vi "count rate.vi"() -> (2 "output waveform":waveform(i32), 3 "Counts per second":i32[](array[numeric])=[0, 39, 50, 53, 43, 50, 43, 47, 49, 37, 40, 55, 56, 54, 41, 52, 42, 50, 55, 55, 45, 36, 58, 52, 48, 47, 54, 50, 64, 44, 52, 51, 34, 52, 46, 42, 50, 45, 40, 42, 45, 40, 42, 59, 53, 48, 43, 37, 28, 32, 29, 31, 30, 44, 40, 33, 48, 33, 36, 38, 41, 31, 35, 37, 38, 40, 40, 22, 25, 37, 35, 33, 39, 39, 33, 33, 30, 28, 35, 32, 21, 45, 30, 25, 33, 21, 30, 28, 34, 17, 24, 19, 24, 27, 32, 30, 18, 28, 28, 22, 18, 23, 28, 33, 21, 18, 24, 20, 30, 26, 27, 17, 19, 22, 18, 21, 16, 20, 20, 19, 18, 22, 22, 22, 22, 22, 25, 24, 16, 20, 12, 21, 17, 24, 14, 24, 11, 13, 19, 21, 18, 13, 11, 13, 10, 15, 12, 12, 18, 12, 18, 18, 14, 11, 17, 16, 10, 11, 22, 18, 17, 10, 10, 10, 14, 17, 11, 8, 11, 13, 7, 10, 14, 13, 16, 13, 8, 9, 11, 10, 10, 4, 10, 10, 8, 13, 10, 9, 16, 13, 11, 10, 4, 7, 7, 8, 7, 6, 7, 10, 8, 9, 12, 13, 7, 11, 11, 0, 11, 9, 7, 6, 11, 10, 1, 11, 5, 4, 10, 9, 8, 5, 6, 11, 9, 8, 3, 10, 6, 7, 8, 7, 5, 7, 6, 8, 9, 9, 8, 9, 8, 6, 6, 10, 7, 4, 7, 8, 2, 9, 9, 10, 8, 7, 9, 3, 4, 7, 4, 5, 8, 4, 6, 6, 9, 3, 8, 8, 7, 5, 10, 4, 7, 2, 9, 9, 6, 3, 3, 4, 4, 2, 5, 3, 2, 4, 8, 8, 3, 5, 1, 6, 3, 1, 4, 5, 6, 7, 2, 5, 3, 3])   [LabVIEW 2014]
uses:
  <vilib>/Platform/TimedLoop/XDataNode/timing_clust.ctl
  <vilib>/Platform/TimedLoop/XDataNode/nitl_modes.ctl
  <vilib>/Platform/TimedLoop/XDataNode/wakeup.ctl
  <vilib>/Waveform/WDTFileIO.llb/ Write Waveform to File.vi
  <vilib>/Utility/file.llb/Write To Spreadsheet File (I64).vi
  <vilib>/platform/TimedLoop/XDataNode/XDataNode.xnode
  <vilib>/Platform/TimedLoop/XDataNode/XDNodeRunTimeDep.lvlib
panel:
  out "Waveform Graph":waveform(i32)(graph)
  in  "Period (ms)":i64=1000
  in  "Total time (sec)":i32=300
  out "counts per second":dbl(knob)=3.0 scale=0.0..100.0
  # "Demo count rate VI for Physics 434"
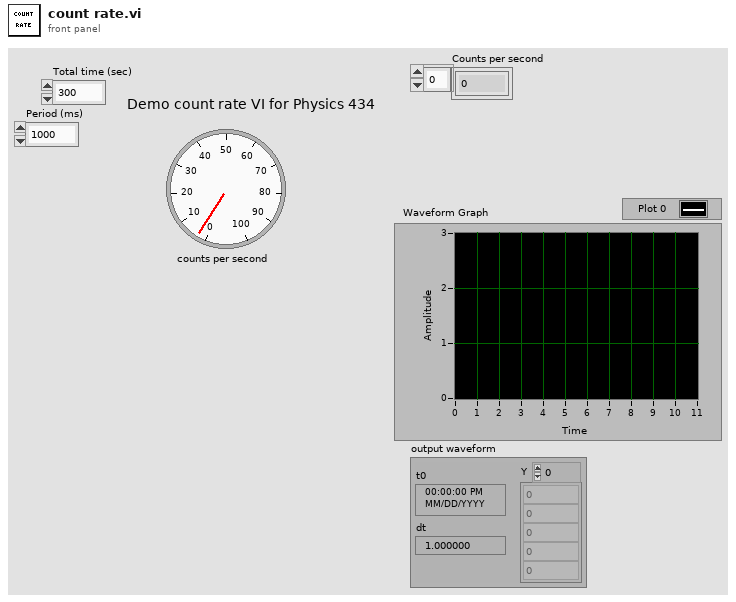
[diagram p1: front panel]
types:
  T1 = typedef "XDNodeRunTimeDep.lvlib/timing_clust.ctl" = cluster{"Expected End [f-1]":u64, "Actual End [f-1]":u64, "Finished Late? [f-1]":bool, "Expected End [i-1]":u64, "Actual End [i-1]":u64, "Finished Late? [i-1]":bool, "Expected Start [i]":u64, "Actual Start [i]":u64, "Expected Start [f]":u64, "Actual Start [f]":u64, "Source Name":string, "Structure Name":string, "Period":i64, "Deadline":i64, "Offset":i64, "Start":i64, "Priority":i32, "Timeout":i32, "Mode":T2, "Wakeup Reason":T3, "Error":errorcluster, "Source Type":string, "Secondary Source Type":string, "Global End Time":u64, "Global Start Time":u64, "Frame Duration":u64, "Iteration Duration":u64, "Assigned CPU":i32, "I/O Scan Engine Mode":u32}
  T2 = typedef "XDNodeRunTimeDep.lvlib/nitl_modes.ctl" = enum32{"No Change", "Process missed periods, maintain original phase", "Discard missed periods, maintain original phase", "Process missed periods, ignore original phase", "Discard missed periods, ignore original phase"}
  T3 = typedef "XDNodeRunTimeDep.lvlib/wakeup.ctl" = enum32{"Normal", "Aborted", "Asynchronous wakeup", "Timing source error", "Timed loop error", "Timeout"}
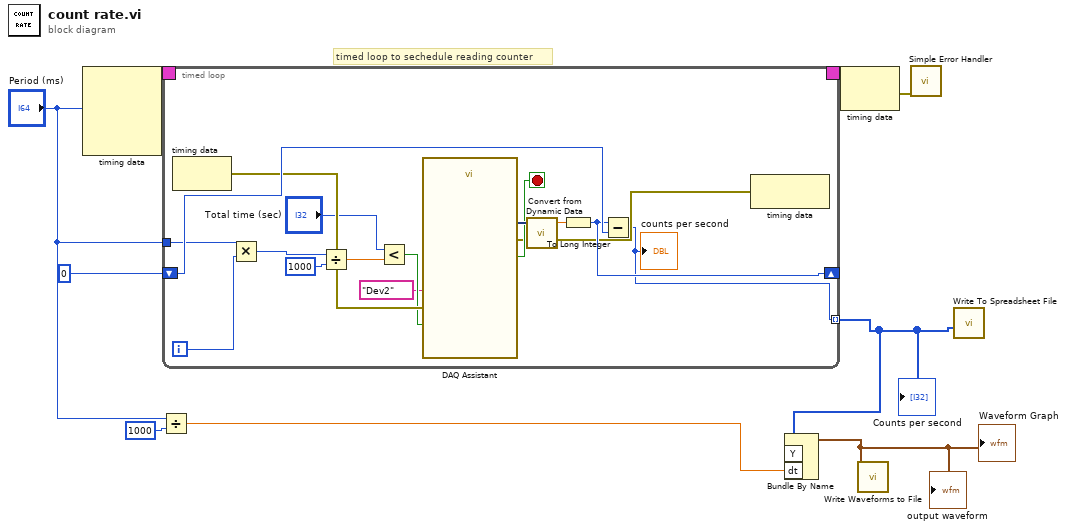
[diagram p0: block diagram]
diagram:
  # "timed loop to sechedule reading counter"
  n1 = node-c288("Period (ms)") -> (w9:T1)  [unwired: 3 in]
  n2 = Divide(x="Period (ms)", y=1000) -> (x/y=w3:dbl)
  n3 = timed-loop {
    timing: w9 -> [_]
    timing-out: [_] -> w8
    tunnel: "Period (ms)" -> [w13]
    shift-right: [w22] -> _
    shift-left: 0 -> [w24]
    tunnel: [w10] -> w2 mode=indexing
    i -> [w12]
    stop <- w23 stop-if-true
    n4 = node-c288() -> (w19:errorcluster)  [unwired: 1 in]
    n5 = Multiply(x=w13, y=w12) -> (x*y=w11:i64)
    n6 = Divide(x=w11, y=1000) -> (x/y=w18:dbl)
    n7 = Less?(x="Total time (sec)", y=w18) -> (x < y?=w15:bool)
    n8 = call "DAQ Assistant"("error in"=w19, "stop (F)"=w15, "device name"=tag "Dev2") -> ("data"=w25:dynamicdata, "stopped"=w23:bool, "error out"=w20:errorcluster)  [unwired: 13 in, 1 out]
    n9 = call "Convert from Dynamic Data"("Dynamic Data Type"=w25) -> ("Scalar"=w21:dbl)  [unwired: 3 in]
    n10 = To Long Integer(number=w21) -> (32bit integer=w22:i32)
    n11 = Subtract(x=w22, y=w24) -> (x-y=w10:i32)
    "counts per second" <- w10
    n12 = node-c288(w20) -> ()  [unwired: 1 out]
  }
  "Counts per second" <- w2
  n13 = Bundle By Name("Y"=w2, "dt"=w3) -> (w1:waveform(i32))  [unwired: 1 in]
  "Waveform Graph" <- w1
  "output waveform" <- w1
  n14 = node-c288(w8) -> (w6:errorcluster)
  n15 = call-poly <vilib>:"Write Waveforms to File.vi"("waveform"=w1) -> ()  [unwired: 9 in, 2 out]
  n16 = call <vilib>:"Simple Error Handler.vi"("error in (no error)"=w6) -> ()  [unwired: 4 in, 5 out]
  n17 = call-poly <vilib>:"Write To Spreadsheet File.vi"("1D data"=w2) -> ()  [unwired: 7 in, 1 out]
